vi "CAN_AI_Time (FPGA).vi"() -> ()   [LabVIEW 2015]
doc: "This example transmits one frame contained in Data Frame every time the Write button is pressed. After building this FPGA VI, you run it using CAN Channel Transmit (Host).vi (not standalone).\n\nThis example assumes the following configuration for CAN 0: Auto Start = True, Listen Only = False, Input Timeout = 10000ms, Output Timeout = 10000ms. The CAN Output node is configured to use an array of U32 for the CAN frame. For more information on configuration, refer to the Help for the NI 9853 CAN module."
uses:
  <vilib>/LabVIEW Targets/FPGA/RIO/nicrio_985x_controls.llb/CAN_IO_SJA1000 Acceptance Filter.ctl
  <vilib>/Platform/TimedLoop/XDataNode/timing_clust.ctl
  <vilib>/Platform/TimedLoop/XDataNode/nitl_modes.ctl
  <vilib>/Platform/TimedLoop/XDataNode/wakeup.ctl
  <vilib>/rvi/Emulation/niFpgaGetClockAttributes.vi
  <vilib>/rvi/Emulation/niFpgaSctlEmulationGetInTimedLoop.vi
  <vilib>/rvi/Emulation/niFpgaEmulationReportErrorSimple.vi
  <vilib>/rvi/eio/common/nirviEmuTemplateMethod_errors.vi
  <vilib>/rvi/interface/RandomDataEmulation/niFpgaRandomDataHandleErrors.vi
  <vilib>/rvi/Emulation/niFpgaCriticalErrorInLSC.vi
  <vilib>/rvi/Emulation/niFpgaProcessEmulError.vi
  <vilib>/rvi/eio/common/nirviEmuTemplatePropertySet_noerrors.vi
  <vilib>/eio/EIONode/EIONode.xnode
  <vilib>/rvi/DataTransferAndStorage/Container/XNode/niFpgaContainer.xnode
  <vilib>/rvi/interface/RandomDataEmulation/nirviRandomDataFpgaReadWriteTemplate.vi
  <vilib>/Platform/TimedLoop/XDataNode/XDataNode.xnode
  <vilib>/eio/EIOPropertyNode/EIOPropertyNode.xnode
  <vilib>/LabVIEW Targets/FPGA/RIO/nicrio_985x_controls.llb/CAN_IO_Frame Array U32.ctl
  <vilib>/rvi/eio/common/nirviEmuTemplatePropertyGet_errors.vi
  <vilib>/rvi/eio/common/nirviEmuTemplatePropertyGet_noerrors.vi
  <vilib>/rvi/eio/common/nirviEmuTemplatePropertySet_errors.vi
  examples copy/Timekeeper/FPGA Timekeeper.lvlib
  <vilib>/Platform/TimedLoop/XDataNode/XDNodeRunTimeDep.lvlib
panel:
  out "FPGA Timekeeper time (ns)":u64
  out "FPGA Timekeeper locked":bool
  out "offset from RT time (ns)":i32
  in  "RT time (ns)":u64
  in  "Rate (uSec)":u32 caption="Count(uSec)"
  out "AI 9205 loop rate":u32
  out "Mod3/AI0":fxp<+/-,26,5>
  out "Mod3/AI1":fxp<+/-,26,5>
  out "Timed Out?":bool
  in  "SJA1000 Filter Code":u32
  in  "SJA1000 Filter Mask":u32
  in  "SJA1000 Filter Mode":T1=enum."Single"
  in  "Set Filter and Start":bool
  out "CAN Frames Pushed":i32
  out "CAN FIFO Full":bool
  out "Actual loop rate CAN":u32
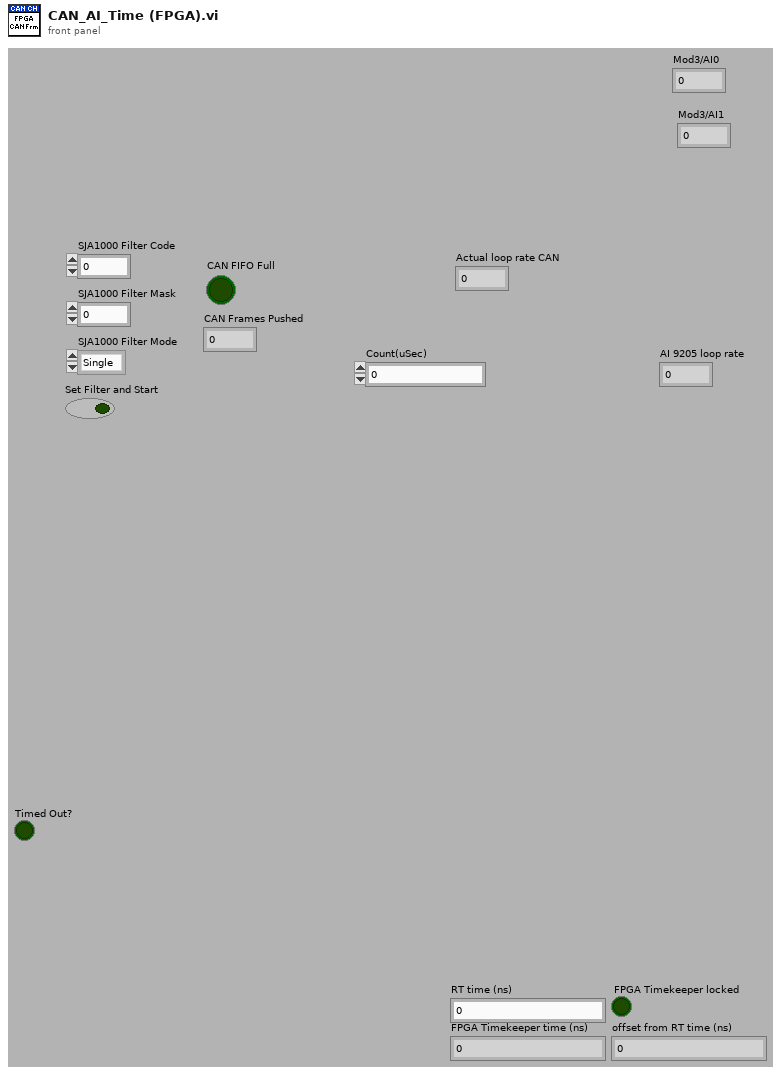
[diagram p1: front panel]
types:
  T1 = typedef "CAN_IO_SJA1000 Acceptance Filter.ctl" = enum8{"Dual", "Single"}
  T2 = typedef "CAN_IO_Frame Array U32.ctl" = u32[]
  T3 = typedef "XDNodeRunTimeDep.lvlib/timing_clust.ctl" = cluster{"Expected End [f-1]":u64, "Actual End [f-1]":u64, "Finished Late? [f-1]":bool, "Expected End [i-1]":u64, "Actual End [i-1]":u64, "Finished Late? [i-1]":bool, "Expected Start [i]":u64, "Actual Start [i]":u64, "Expected Start [f]":u64, "Actual Start [f]":u64, "Source Name":string, "Structure Name":string, "Period":i64, "Deadline":i64, "Offset":i64, "Start":i64, "Priority":i32, "Timeout":i32, "Mode":T4, "Wakeup Reason":T5, "Error":errorcluster, "Source Type":string, "Secondary Source Type":string, "Global End Time":u64, "Global Start Time":u64, "Frame Duration":u64, "Iteration Duration":u64, "Assigned CPU":i32, "I/O Scan Engine Mode":u32}
  T4 = typedef "XDNodeRunTimeDep.lvlib/nitl_modes.ctl" = enum32{"No Change", "Process missed periods, maintain original phase", "Discard missed periods, maintain original phase", "Process missed periods, ignore original phase", "Discard missed periods, ignore original phase"}
  T5 = typedef "XDNodeRunTimeDep.lvlib/wakeup.ctl" = enum32{"Normal", "Aborted", "Asynchronous wakeup", "Timing source error", "Timed loop error", "Timeout"}
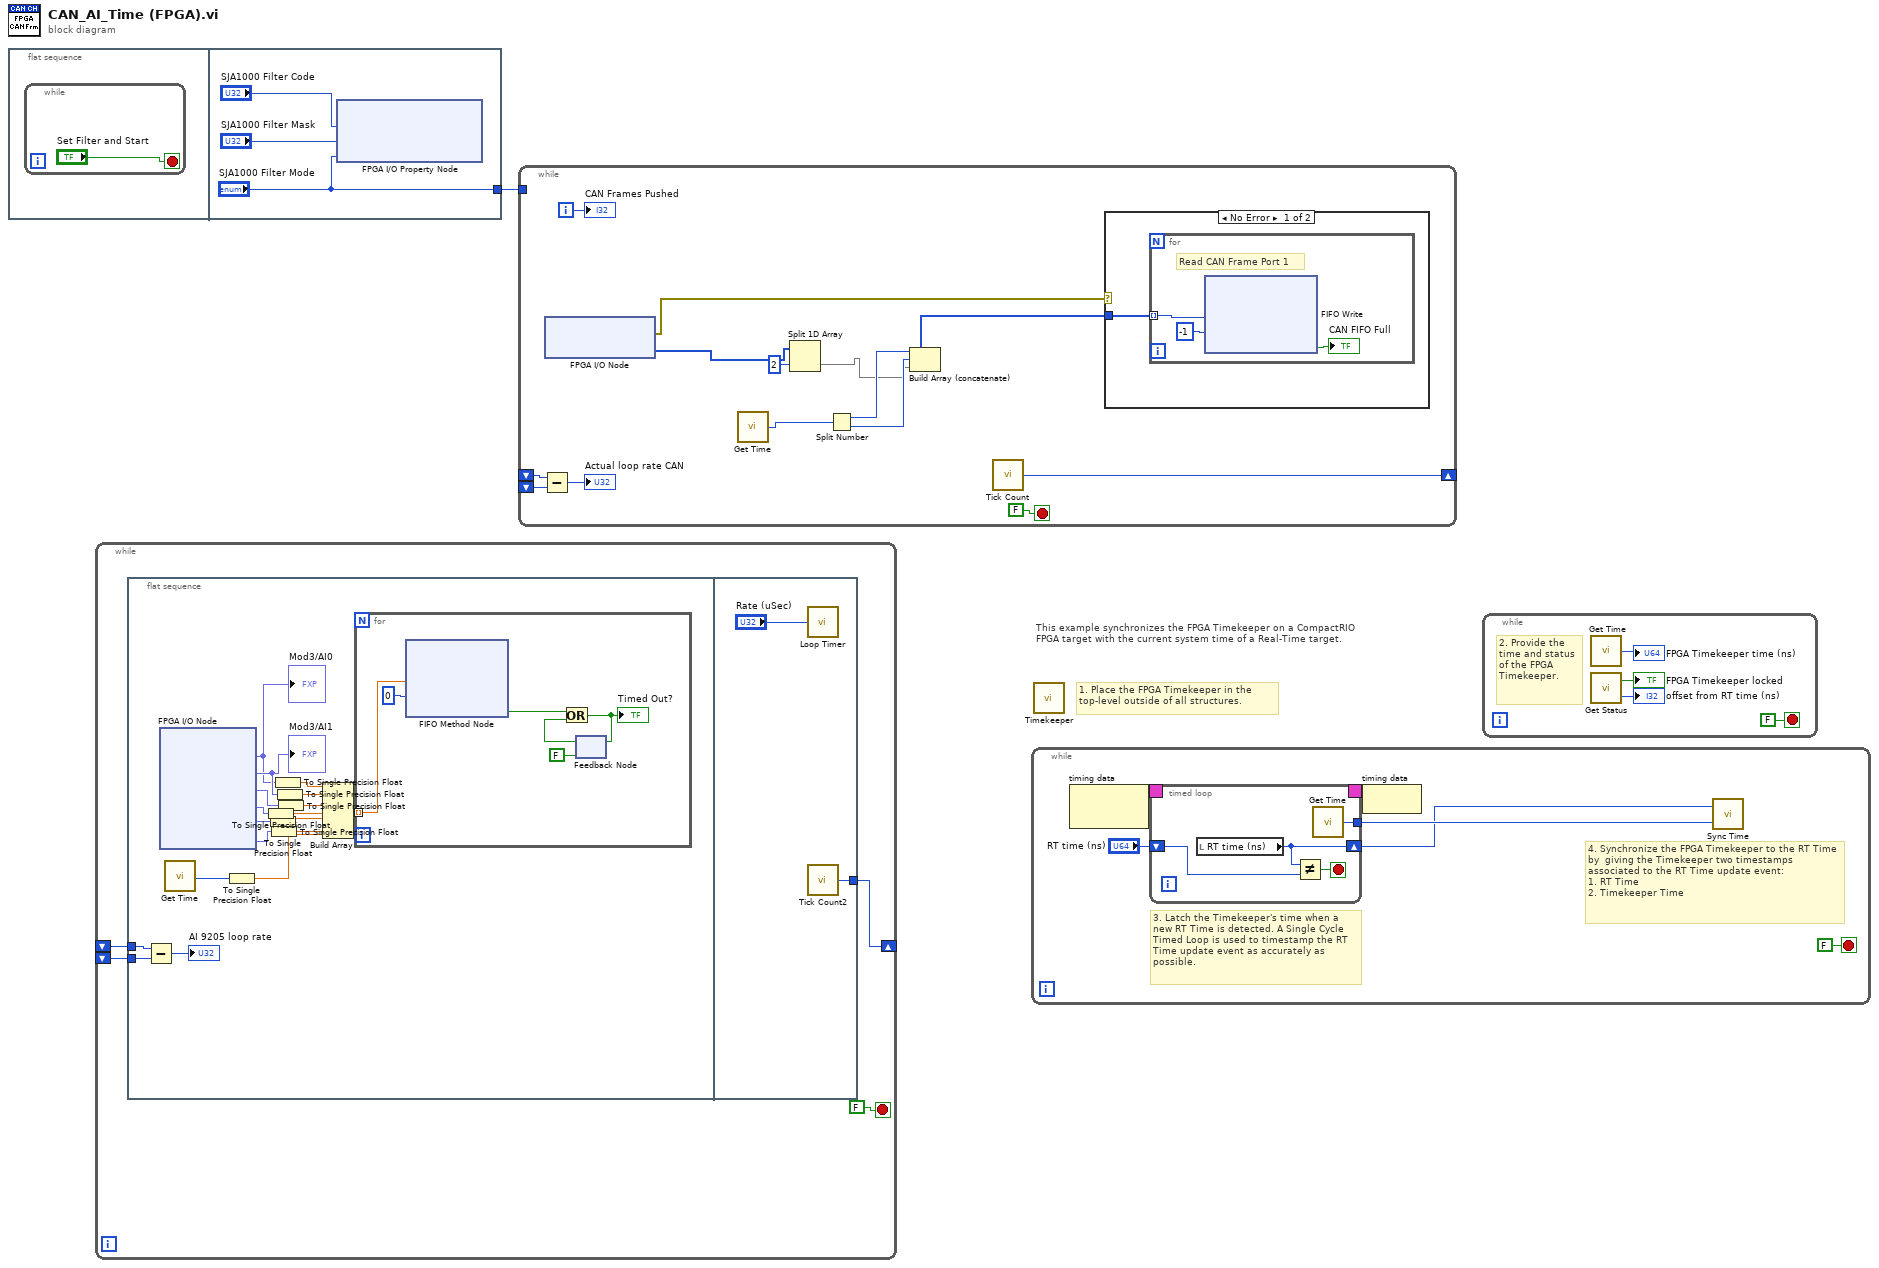
[diagram p0: block diagram]
diagram:
  # "This example synchronizes the FPGA Timekeeper on a CompactRIO FPGA target with the current system time of a Real-Time target."
  # "1. Place the FPGA Timekeeper in the top-level outside of all structures."
  n1 = flat-sequence {
    tunnel: ["SJA1000 Filter Mode"] -> w1
    frame #0 {
      n2 = while {
        stop <- "Set Filter and Start" stop-if-true
      }
    }
    frame #1 {
      n3 = xnode "FPGA I/O Property Node"("SJA1000 Filter Code"="SJA1000 Filter Code", "SJA1000 Filter Mask"="SJA1000 Filter Mask", "SJA1000 Filter Mode"="SJA1000 Filter Mode") -> ()  [unwired: 1 in, 1 out]
    }
  }
  n4 = while {
    shift-right: [w8] -> _
    shift-left: _ -> [w7]
    shift-left: _ -> [w6]
    stop <- FALSE stop-if-true
    n5 = flat-sequence {
      tunnel: w7 -> [w27]
      tunnel: w6 -> [w26]
      tunnel: [w34] -> w8
      frame #0 {
        n6 = Subtract(x=w27, y=w26) -> (x-y=→"AI 9205 loop rate":u32)
        n7 = xnode "FPGA I/O Node"() -> ("Mod3/AI0"=w12:fxp<+/-,26,5>, "Mod3/AI1"=w13:fxp<+/-,26,5>, "Mod3/AI2"=w15:fxp<+/-,26,5>, "Mod3/AI3"=w19:fxp<+/-,26,5>, "Mod3/AI4"=w16:fxp<+/-,26,5>, "Mod3/AI5"=w21:fxp<+/-,26,5>)  [unwired: 6 in, 6 out]
        "Mod3/AI0" <- w12
        "Mod3/AI1" <- w13
        n8 = call "Get Time.vi"() -> ("time (ns)"=w23:u64)
        n9 = To Single Precision Float(number=w23) -> (single precision float=w22:sgl)
        n10 = To Single Precision Float(number=w19) -> (single precision float=w18:sgl)
        n11 = To Single Precision Float(number=w16) -> (single precision float=w17:sgl)
        n12 = To Single Precision Float(number=w21) -> (single precision float=w20:sgl)
        n13 = To Single Precision Float(number=w12) -> (single precision float=w11:sgl)
        n14 = To Single Precision Float(number=w13) -> (single precision float=w10:sgl)
        n15 = To Single Precision Float(number=w15) -> (single precision float=w14:sgl)
        n16 = Build Array(w11, w10, w14, w18, w17, w20, w22) -> (w24:sgl[])
        n17 = for {
          tunnel: w24 -> [w33] mode=indexing
          n18 = xnode ("FIFO Method Node")("Element"=w33, "Timeout"=0) -> ("Timed Out?"=w31:bool)  [unwired: 1 in, 1 out]
          n19 = feedback #1(FALSE) -> (w30:bool)
          n20 = Or(x=w31, y=w30) -> (x .or. y?=w29:bool)
          "Timed Out?" <- w29
          n21 = feedback-in #1(w29) -> ()
        }
      }
      frame #1 {
        n22 = call "Loop Timer"("Count(uSec)"="Rate (uSec)") -> ()  [unwired: 1 out]
        n23 = call "Tick Count2"() -> ("Tick Count(uSec)"=w34:u32)
      }
    }
  }
  n24 = while {
    tunnel: w1 -> [_]
    shift-right: [w46] -> _
    shift-left: _ -> [w44]
    shift-left: _ -> [w43]
    i -> [w48]
    stop <- FALSE stop-if-true
    n25 = Subtract(x=w44, y=w43) -> (x-y=→"Actual loop rate CAN":u32)
    n26 = xnode "FPGA I/O Node"() -> ("error out"=w47:errorcluster, "Mod1/CAN0"=w42:T2)  [unwired: 2 in, 1 out]
    n27 = call "Get Time.vi"() -> ("time (ns)"=w40:u64)
    n28 = Split 1D Array(array=w42, index=2) -> (second subarray=w37:T2)  [unwired: 1 out]
    n29 = Split Number(x=w40) -> (hi(x)=w39:u32, lo(x)=w38:u32)
    n30 = Build Array (concatenate)(w39, w38, w37) -> (w41:u32[])
    n31 = call "Tick Count"() -> ("Tick Count(uSec)"=w46:u32)
    n32 = case shown="No Error" w47 {
      tunnel: w41 -> [w50 _]
      frame No Error {
        n33 = for {
          tunnel: w50 -> [w51] mode=indexing
          # "Read CAN Frame Port 1"
          n34 = xnode ("FIFO Write")("Element"=w51, "Timeout"=-1) -> ("Timed Out?"=→"CAN FIFO Full":bool)  [unwired: 1 in, 1 out]
        }
      }
      frame Error {
      }
    }
    "CAN Frames Pushed" <- w48
  }
  n35 = while {
    stop <- FALSE stop-if-true
    # "3. Latch the Timekeeper's time when a new RT Time is detected. A Single Cycle Timed Loop is used to timestamp the RT Time update event as accurately as possible."
    # "4. Synchronize the FPGA Timekeeper to the RT Time by  giving the Timekeeper two timestamps associated to the RT Time update event:\n1. RT Time\n2. Timekeeper Time"
    n36 = node-c288() -> (w59:T3)  [unwired: 1 in]
    n37 = timed-loop {
      timing: w59 -> [_]
      timing-out: [_] -> w58
      shift-right: [w60] -> w54
      shift-left: "RT time (ns)" -> [w61]
      tunnel: [w63] -> w57
      stop <- w62 stop-if-true
      n38 = local read "RT time (ns)"() -> (w60:u64)
      n39 = Not Equal?(x=w60, y=w61) -> (x != y?=w62:bool)
      n40 = call "Get Time.vi"() -> ("time (ns)"=w63:u64)
    }
    n41 = node-c288(w58) -> ()
    n42 = call "Sync Time.vi"("FPGA Timekeeper time (ns)"=w57, "time reference time (ns)"=w54) -> ()
  }
  n43 = call "Timekeeper.vi"() -> ()  [unwired: 12 in]
  n44 = while {
    stop <- FALSE stop-if-true
    # "2. Provide the time and status of the FPGA Timekeeper."
    n45 = call "Get Time.vi"() -> ("time (ns)"=→"FPGA Timekeeper time (ns)":u64)
    n46 = call "Get Status.vi"() -> ("FPGA Timekeeper locked"=→"FPGA Timekeeper locked":bool, "offset from time reference"=→"offset from RT time (ns)":i32)
  }
